vi "initialize Session Data.vi"(0 "Session in":refnum<class "Configurations.lvclass">, 11 "error in":errorcluster) -> (4 "Session out":refnum<class "Configurations.lvclass">, 15 "error out":errorcluster)   [LabVIEW 2016, in "Configurations.lvlib" / "Configurations.lvclass"]
uses:
  Configurations.lvclass
  <vilib>/Utility/config.llb/NI_LVConfig.lvlib
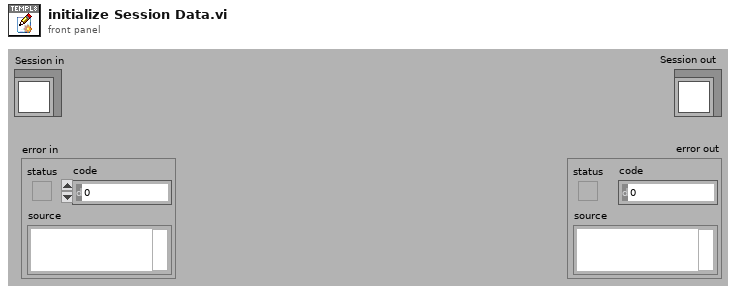
[diagram p1: front panel]
types:
  T1 = typedef "NI_LVConfig.lvlib/Config Data RefNum.ctl" = refnum<k1>
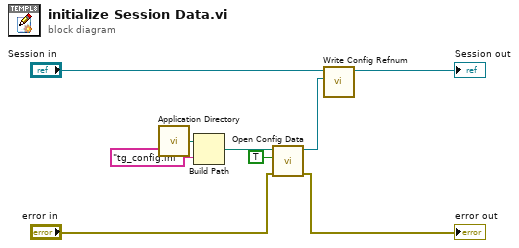
[diagram p0: block diagram]
diagram:
  n1 = call <vilib>:"Application Directory.vi"() -> ("Application Directory"=w6:path)
  n2 = Build Path(base path=w6, name or relative path="tg_config.ini") -> (appended path=w8:path)
  n3 = call <vilib>:"Open Config Data.vi"("error in (no error)"="error in", "create file if necessary (T)"=TRUE, "configuration file path"=w8) -> ("error out"=→"error out":errorcluster, "refnum"=w4:T1)  [unwired: 6 in, 1 out]
  n4 = call-dynamic "Write Config Refnum.vi"("config data"=w4, "Configurations in"="Session in") -> ("Configurations out"=→"Session out":refnum<class "Configurations.lvclass">)  [unwired: 9 in]
